vi "create_ID.vi"(8 "error in (no error)":errorcluster) -> (0 "error out":errorcluster, 2 "ID":dbl)   [LabVIEW 2010, in "PointCollection.lvclass"]
uses:
  PointCollection.lvclass
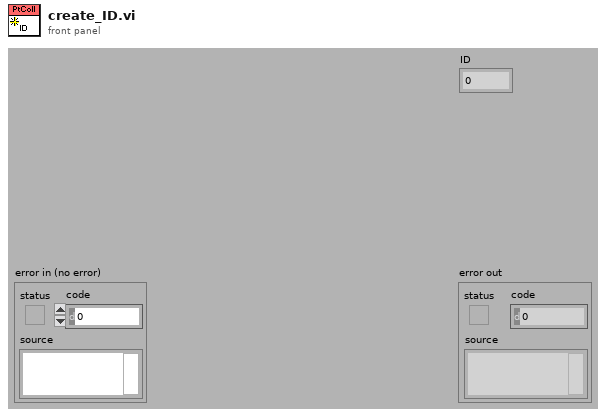
[diagram p1: front panel]
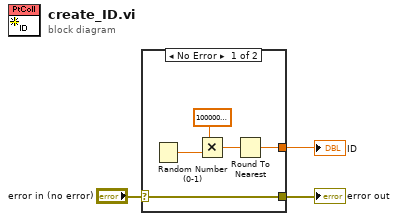
[diagram p0: block diagram]
diagram:
  n1 = case shown="No Error" "error in (no error)" {
    selector: "error in (no error)" -> [w8 w9]
    tunnel: [w8 w9] -> w2
    tunnel: [w4 _] -> w1
    frame No Error {
      n2 = Random Number (0-1)() -> (number: 0 to 1=w7:dbl)
      n3 = Multiply(x=100000000000000.0, y=w7) -> (x*y=w5:dbl)
      n4 = Round To Nearest(number=w5) -> (nearest integer value=w4:dbl)
    }
    frame Error {
    }
  }
  "error out" <- w2
  "ID" <- w1
